vi "MM9.contents.vi"() -> ()   [LabVIEW 2014, in "MM9.lvlib"]
doc: "loads all VIs into memory - required for building an application"
uses:
  MM9.lvlib
panel:
  out "error out":errorcluster
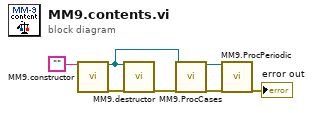
[diagram p0: block diagram]
diagram:
  n1 = call "MM9.constructor.vi"("name"="") -> ("i ref out"=w5:refnum<vi>, "error out"=w4:errorcluster)  [unwired: 16 in, 1 out]
  n2 = call "MM9.destructor.vi"("i ref in"=w5, "error in (no error)"=w4) -> ("error out"=w3:errorcluster)  [unwired: 17 in]
  n3 = call "MM9.ProcCases.vi"("i ref in"=w5, "error in (no error)"=w3) -> ("i ref out"=w6:refnum<vi>, "error out"=w2:errorcluster)  [unwired: 15 in, 1 out]
  n4 = call "MM9.ProcPeriodic.vi"("i ref in"=w6, "error in (no error)"=w2) -> ("error out"=→"error out":errorcluster)  [unwired: 15 in, 2 out]
